vi "Create Arbitrary Waveform.vi"(7 "Arbitrary Waveform Name (0: USER1)":u16(ring) items=["USER1", "USER2", "USER3", "USER4"], 8 "error in (no error)":errorcluster, 9 "Arbitrary Waveform Data":dbl[](array[numeric]), 10 "Edit Memory (0: Edit Memory)":i32(ring) items=["Edit Memory", "Edit Memory 1", "Edit Memory 2"], 11 "VISA resource name":refnum<visa-resource-name>) -> (0 "error out":errorcluster, 3 "VISA resource name out":refnum<visa-resource-name>)   [LabVIEW 2015, in "Tektronix AFG 3000 Series.lvlib"]
doc: "Creates and saves an arbitrary waveform in edit memory. \n\n<B>Note:</B>\n\nCreates an arbitrary waveform in the specified edit memory and because of this, the waveform will remain stored on the instrument until deleted. If any sensitive information is contained in the arbitrary waveform, it is recommended that the waveform be deleted when finished."
uses:
  Tektronix AFG 3000 Series.lvlib
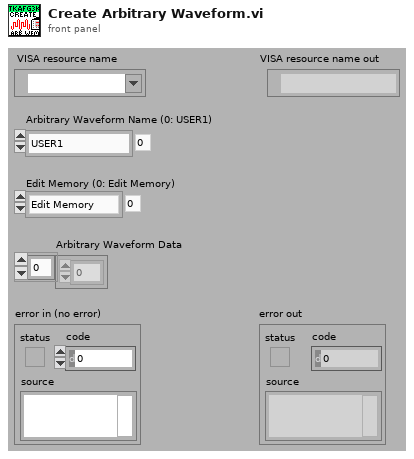
[diagram p1: front panel]
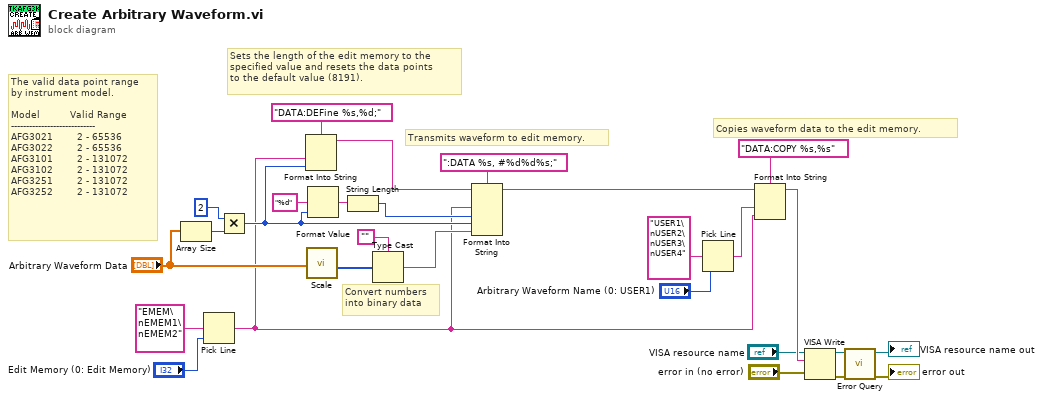
[diagram p0: block diagram]
diagram:
  # "The valid data point range \nby instrument model. \n\nModel          Valid Range\n----------------------------\nAFG3021        2 - 65536\nAFG3022        2 - 65536\nAFG3101        2 - 131072\nAFG3102        2 - 131072\nAFG3251        2 - 131072\nAFG3252        2 - 131072"
  # "Convert numbers\ninto binary data"
  # "Transmits waveform to edit memory."
  # "Sets the length of the edit memory to the \nspecified value and resets the data points \nto the default value (8191)."
  # "Copies waveform data to the edit memory."
  n1 = Array Size(array="Arbitrary Waveform Data") -> (size(s)=w21:i32)
  n2 = Pick Line(multi-line string="EMEM\nEMEM1\nEMEM2" ("format string"), line index="Edit Memory (0: Edit Memory)") -> (output string=w1:string)  [unwired: 1 in]
  n3 = Multiply(x=2, y=w21) -> (x*y=w5:i32)
  n4 = Format Into String(format string="DATA:DEFine %s,%d;", w1, w5) -> (resulting string=w14:string)  [unwired: 2 in, 1 out]
  n5 = call "Scale.vi"("Waveform Data"="Arbitrary Waveform Data") -> ("Scaled Waveform Data"=w9:u16[])  [unwired: 10 in]
  n6 = Format Value(format string="%d", value (0)=w5) -> (output string=w12:string)  [unwired: 1 in]
  n7 = String Length(string=w12) -> (length=w4:i32)
  n8 = Type Cast(type="", x=w9) -> (*(type *) &x=w6:string)
  n9 = Format Into String(format string=":DATA %s, #%d%d%s;", initial string=w14, w1, w4, w5, w6) -> (resulting string=w11:string)  [unwired: 1 in, 1 out]
  n10 = Pick Line(multi-line string="USER1\nUSER2\nUSER3\nUSER4", line index="Arbitrary Waveform Name (0: USER1)") -> (output string=w17:string)  [unwired: 1 in]
  n11 = Format Into String(format string="DATA:COPY %s,%s", initial string=w11, w17, w1) -> (resulting string=w16:string)  [unwired: 1 in, 1 out]
  n12 = VISA Write(VISA resource name="VISA resource name", write buffer=w16, error in (no error)="error in (no error)") -> (VISA resource name out=w27:refnum<visa-resource-name>, error out=w28:errorcluster)  [unwired: 1 out]
  n13 = call "Error Query.vi"("error in (no error)"=w28, "VISA resource name"=w27) -> ("error out"=→"error out":errorcluster, "VISA resource name out"=→"VISA resource name out":refnum<visa-resource-name>)  [unwired: 6 in, 2 out]
